vi "Add Child at Index.vi"(4 "Insertion Index":i32=-1, 6 "Unique ID":string, 11 "Linked List Definition in":refnum<class "Linked List Definition.lvclass">) -> (3 "Linked List Definition out":refnum<class "Linked List Definition.lvclass">)   [LabVIEW 2020, in "Linked Lists.lvlib" / "Linked List Definition.lvclass"]
uses:
  <vilib>/gpm_packages/@cs/linked-list/Source/Linked List/Linked List Definition/Linked List Definition.lvclass
  <vilib>/gpm_packages/@cs/linked-list/Source/Linked List/Linked List Definition/Linked List Definition.lvclass/Linked List Definition.ctl
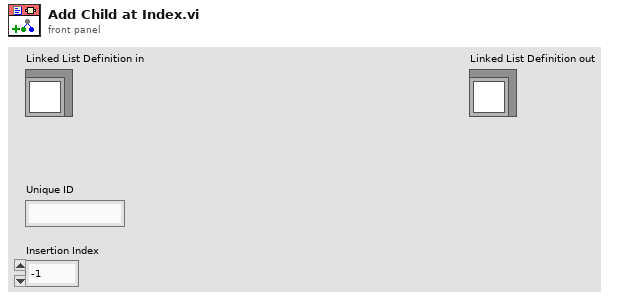
[diagram p1: front panel]
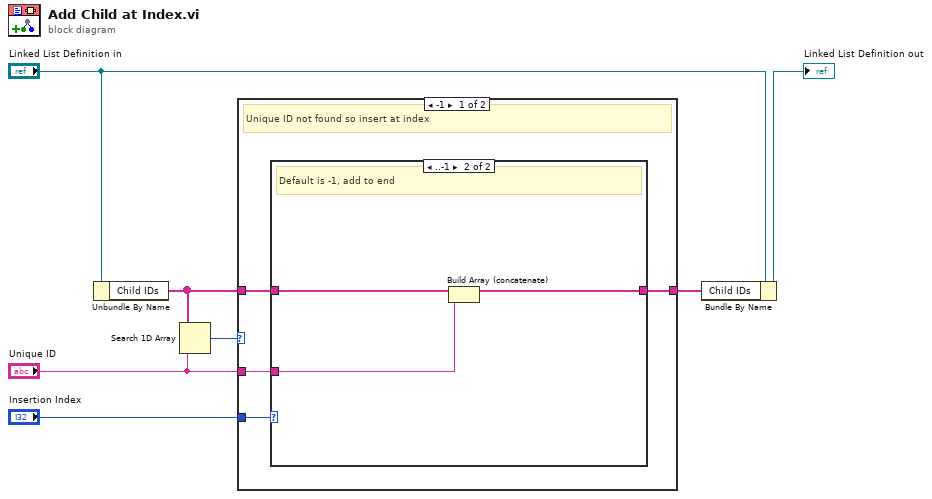
[diagram p0: block diagram]
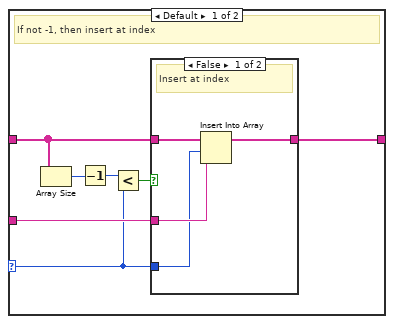
[diagram p2: hidden frame]
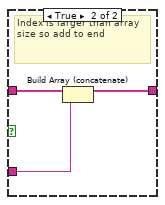
[diagram p3: hidden frame]
diagram:
  n1 = Unbundle By Name("Linked List Definition in") -> ("Child IDs"=w6:string[])
  n2 = Search 1D Array(1D array=w6, element="Unique ID") -> (index of element=w7:i32)  [unwired: 1 in]
  n3 = case shown="-1" w7 {
    tunnel: w6 -> [w11 w29]
    tunnel: "Unique ID" -> [w10 _]
    tunnel: [w9 w29] -> w1
    tunnel: "Insertion Index" -> [w8 _]
    frame -1 {
      # "Unique ID not found so insert at index"
      n4 = case shown="..-1" w8 {
        selector: w8 -> [w13 _]
        tunnel: w11 -> [w14 w28]
        tunnel: w10 -> [w17 w27]
        tunnel: [w18 w26] -> w9
        frame Default {
          # "If not -1, then insert at index"
          n5 = Array Size(array=w14) -> (size(s)=w16:i32)
          n6 = Decrement(x=w16) -> (x-1=w15:i32)
          n7 = Less?(x=w15, y=w13) -> (x < y?=w12:bool)
          n8 = case shown="False" w12 {
            tunnel: [w22 w24] -> w18
            tunnel: w17 -> [w21 w23]
            tunnel: w14 -> [w20 w25]
            tunnel: w13 -> [w19 _]
            frame False {
              # "Insert at index"
              n9 = Insert Into Array(array=w20, index=w19, new element=w21) -> (w22:string[])
            }
            frame True {
              # "Index is larger than array size so add to end"
              n10 = Build Array (concatenate)(w25, w23) -> (w24:string[])
            }
          }
        }
        frame ..-1 {
          # "Default is -1, add to end"
          n11 = Build Array (concatenate)(w28, w27) -> (w26:string[])
        }
      }
    }
    frame Default {
      # "Unique ID already exists"
    }
  }
  n12 = Bundle By Name(cluster="Linked List Definition in", "Child IDs"=w1) -> (→"Linked List Definition out":refnum<class "Linked List Definition.lvclass">)
